vi "Distance Sensor-Remote.vi"() -> (16 "Distance":i32)   [LabVIEW 2009]
uses:
  <vilib>/NXT/Block Support/NXT_InputPort.ctl
  <vilib>/NXT/Subs/LVHSConnector.ctl
  <vilib>/NXT/Dual Mode Library/Display/drawText.vi
panel:
  out "NXT dup":T1={"error"={"status"=FALSE, "code"=0, "source"=""}, "address"="", "NXT #"=-1, "Show Error"=TRUE} caption="NXT"
  in  "NXT":T1={"error"={"status"=FALSE, "code"=0, "source"=""}, "address"="", "NXT #"=-1, "Show Error"=TRUE}
  in  "Input Port":T2 items=["Port 1", "Port 2", "Port 3", "Port 4"]
  # "mindsensors.com\nCopyright (c) 2009 by mindsensors.com\nEmail: info (<at>) mindsensors (<dot>) com\n\nThis program is free software. You can redistribute it and/or modify\nit under the terms of the GNU General Public License as published by\nthe Free Software Foundation; version 3 of the License.\nRead the license at: http://www.gnu.org/licenses/gpl.txt"
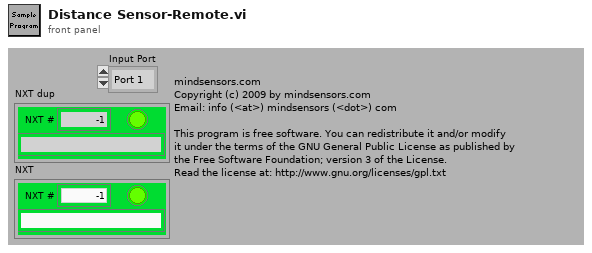
[diagram p1: front panel]
types:
  T1 = typedef "LVHSConnector.ctl" = cluster{"error":errorcluster, "address":string, "NXT #":i32, "Show Error":bool}
  T2 = typedef "NXT_InputPort.ctl" = u8
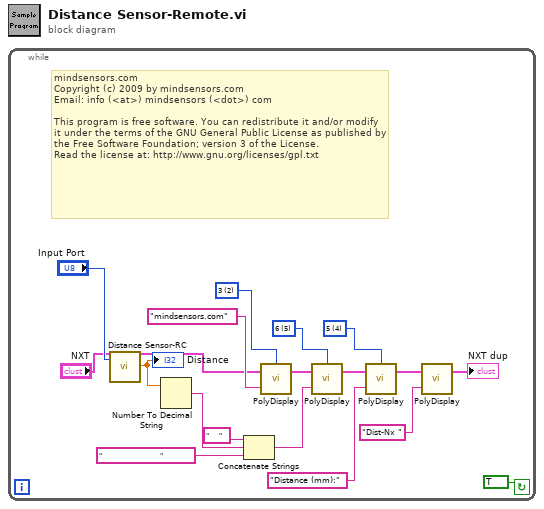
[diagram p0: block diagram]
diagram:
  n1 = while {
    stop <- TRUE continue-if-true
    w10 = i16 4 items=["1", "2", "3", "4", "5", "6", "7", "8"] ("Line")
    w11 = i16 5 items=["1", "2", "3", "4", "5", "6", "7", "8"] ("Line")
    w13 = i16 2 items=["1", "2", "3", "4", "5", "6", "7", "8"] ("Line")
    # "mindsensors.com\nCopyright (c) 2009 by mindsensors.com\nEmail: info (<at>) mindsensors (<dot>) com\n\nThis program is free software. You can redistribute it and/or modify\nit under the terms of the GNU General Public License as published by\nthe Free Software Foundation; version 3 of the License.\nRead the license at: http://www.gnu.org/licenses/gpl.txt"
    n2 = call "Distance Sensor-RC.vi"("NXT"="NXT", "Input Port"="Input Port") -> ("NXT dup"=w5:T1, "Distance Value"=w19:ext)  [unwired: 23 in, 1 out]
    "Distance" <- w19
    n3 = Number To Decimal String(number=w19) -> (decimal integer string=w16:string)  [unwired: 1 in]
    n4 = Concatenate Strings("     " ("string"), w16, "                             " ("string")) -> (w8:string)
    n5 = call-poly <vilib>:"PolyDisplay.vi"("Text"="mindsensors.com", "NXT"=w5, "Line"=w13) -> ("NXT"=w4:T1)  [unwired: 1 in]
    n6 = call-poly <vilib>:"PolyDisplay.vi"("Text"=w8, "NXT"=w4, "Line"=w11) -> ("NXT"=w3:T1)  [unwired: 1 in]
    n7 = call-poly <vilib>:"PolyDisplay.vi"("Text"="Distance (mm):", "NXT"=w3, "Line"=w10) -> ("NXT"=w2:T1)  [unwired: 1 in]
    n8 = call-poly <vilib>:"PolyDisplay.vi"("Text"="Dist-Nx ", "NXT"=w2) -> ("NXT"=→"NXT dup":T1)  [unwired: 2 in]
  }
